vi "IOScan_SetFPSizeToMinimum.vi"(8 "error in":errorcluster, 11 "VI in":refnum<vi>) -> (0 "error out":errorcluster, 3 "VI out":refnum<vi>)   [LabVIEW 2016]
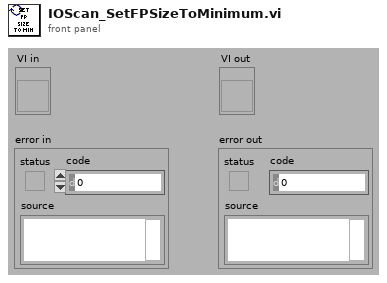
[diagram p1: front panel]
types:
  T1 = typedef "LVPointTypeDef.ctl" = cluster{"Horizontal":i16, "Vertical":i16}
  T2 = typedef "LVRectTypeDef.ctl" = cluster{"Left":i16, "Top":i16, "Right":i16, "Bottom":i16}
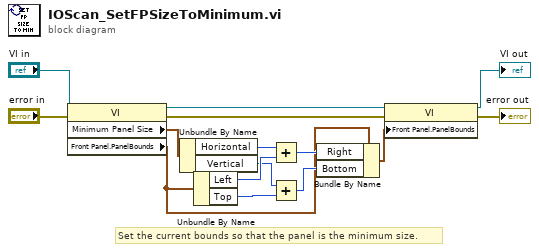
[diagram p0: block diagram]
diagram:
  # "Set the current bounds so that the panel is the minimum size."
  n1 = property class="VI"(reference="VI in", error in="error in") -> (reference out=w2:refnum<vi>, error out=w3:errorcluster, "Minimum Panel Size"=w4:T1, "Front Panel.PanelBounds"=w5:T2)
  n2 = Unbundle By Name(w4) -> ("Horizontal"=w7:i16, "Vertical"=w8:i16)
  n3 = Unbundle By Name(w5) -> ("Left"=w9:i16, "Top"=w10:i16)
  n4 = Add(x=w7, y=w9) -> (x+y=w11:i16)
  n5 = Add(x=w8, y=w10) -> (x+y=w12:i16)
  n6 = Bundle By Name(cluster=w5, "Right"=w11, "Bottom"=w12) -> (w6:T2)
  n7 = property class="VI"(reference=w2, error in=w3, "Front Panel.PanelBounds"=w6) -> (reference out=→"VI out":refnum<vi>, error out=→"error out":errorcluster)
